vi "Realsense Cam Stream Restart.vi"(8 "error in (no error)":errorcluster, 10 "Stream Config":T1={"Stream Type"=enum."Color", "Resolution"=27} {"Resolution" items=["424 x 240 @6fps", "424 x 240 @15fps", "424 x 240 @30fps", "424 x 240 @60fps", "424 x 240 @90fps", "480 x 270 @6fps", "480 x 270 @15fps", "480 x 270 @30fps", "480 x 270 @60fps", "480 x 270 @90fps", "640 x 360 @6fps", "640 x 360 @15fps", "640 x 360 @30fps", "640 x 360 @60fps", "640 x 360 @90fps", "640 x 480 @6fps", "640 x 480 @15fps", "640 x 480 @30fps", "640 x 480 @60fps", "640 x 480 @90fps", "848 x 100 @100fps", "848 x 480 @6fps", "848 x 480 @15fps", "848 x 480 @30fps", "848 x 480 @60fps", "848 x 480 @90fps", "1280 x 720 @6fps", "1280 x 720 @15fps", "1280 x 720 @30fps", "1280 x 800 @15fps", "1280 x 800 @30fps"]}, 11 "Realsense Cam in":refnum<class "Realsense Cam.lvclass">) -> (0 "error out":errorcluster, 3 "Realsense Cam out":refnum<class "Realsense Cam.lvclass">)   [LabVIEW 2018, in "Realsense Cam.lvclass"]
uses:
  Realsense Cam.lvclass
  Private/Stream Config STYP.ctl
  Private/Stream Types Enum STYP.ctl
  Realsense Cam.lvclass/Realsense Cam.ctl
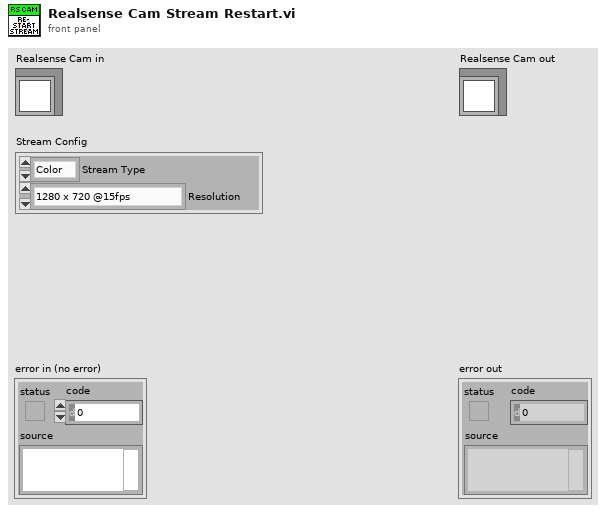
[diagram p1: front panel]
types:
  T1 = typedef "Realsense Cam.lvclass/Stream Config STYP.ctl" = cluster{"Stream Type":T2, "Resolution":u16}
  T2 = typedef "Realsense Cam.lvclass/Stream Types Enum STYP.ctl" = enum16{"Depth", "Left IR", "Left IR Unrectified", "Right IR", "Right IR Unrectified", "Color", "RGB Ext."}
  T3 = cluster{"Depth?":bool, "Left IR?":bool, "Left IR Unrectified?":bool, "Right IR?":bool, "Right IR Unrectified?":bool, "Color?":bool, "RGB Ext.?":bool}
  T4 = typedef "Realsense Cam.lvclass/Activated Stream STYP.ctl" = cluster{"Stream Config":T1, "Profile Handle":u64, "Stream":T5}
  T5 = typedef "Realsense Cam.lvclass/Stream STYP.ctl" = cluster{"Strings":string[], "Intrinsics":cluster{"width":i32, "height":i32, "fps":i32, "Profile":u64, "ppx":sgl, "ppy":sgl, "fx":sgl, "fy":sgl, "model":u32}[], "Current Data":T6}
  T6 = typedef "Realsense Cam.lvclass/Stream Frame Data STYP.ctl" = cluster{"Depths":sgl[][], "Bytes":u8[], "16-Bit IR":u16[], "Height":i32, "Width":i32}
  T7 = cluster{"Status[0]":bool, "Status[1]":bool, "Status[2]":bool, "Status[3]":bool, "Status[4]":bool, "Status[5]":bool, "Status[6]":bool}
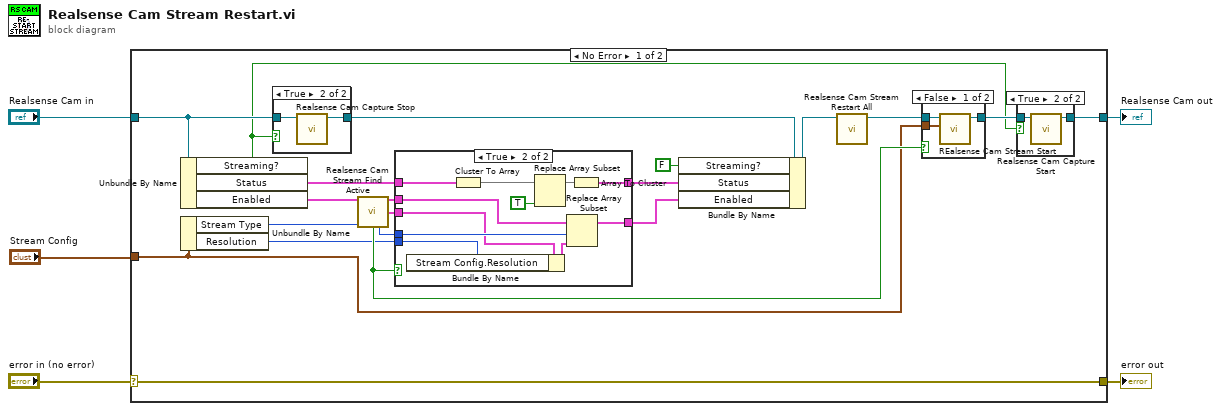
[diagram p0: block diagram]
diagram:
  n1 = case shown="No Error" "error in (no error)" {
    selector: "error in (no error)" -> [w24 w49]
    tunnel: [w24 w49] -> w4
    tunnel: [w7 w48] -> w2
    tunnel: "Realsense Cam in" -> [w19 w48]
    tunnel: "Stream Config" -> [w9 _]
    frame No Error {
      n2 = Unbundle By Name(w19) -> ("Streaming?"=w6:bool, "Status"=w23:T3, "Enabled"=w21:T4[])
      n3 = Unbundle By Name(w9) -> ("Stream Type"=w12:T2, "Resolution"=w11:u16)
      n4 = case shown="True" w6 {
        tunnel: w19 -> [w32 w34]
        tunnel: [w32 w33] -> w16
        frame False {
        }
        frame True {
          n5 = call-dynamic "Realsense Cam Capture Stop.vi"("Realsense Cam in"=w34) -> ("Realsense Cam out"=w33:refnum<class "Realsense Cam.lvclass">)  [unwired: 8 in, 2 out]
        }
      }
      n6 = call "Realsense Cam Stream Find Active.vi"("Streams"=w21, "Stream Types"=w12) -> ("Activated Stream"=w22:T4, "Found?"=w17:bool, "Index"=w20:i32)  [unwired: 11 in]
      n7 = case shown="True" w17 {
        tunnel: w23 -> [w36 w47]
        tunnel: w22 -> [_ w39]
        tunnel: w21 -> [w35 w43]
        tunnel: w20 -> [_ w42]
        tunnel: [w36 w41] -> w14
        tunnel: [w35 w40] -> w10
        tunnel: w11 -> [_ w37]
        frame False {
        }
        frame True {
          n8 = Bundle By Name(cluster=w39, "Stream Config.Resolution"=w37) -> (w38:T4)
          n9 = Cluster To Array(cluster=w47) -> (array=w46:bool[])
          n10 = Replace Array Subset(array=w46, new element=TRUE ("new element/subarray")) -> (w44:bool[])  [unwired: 1 in]
          n11 = Replace Array Subset(array=w43, new element=w38, index=w42) -> (w40:T4[])
          n12 = Array To Cluster(array=w44) -> (cluster=w41:T7)
        }
      }
      n13 = Bundle By Name(cluster=w16, "Streaming?"=FALSE ("Stream Data.Started?"), "Status"=w14, "Enabled"=w10) -> (w15:refnum<class "Realsense Cam.lvclass">)
      n14 = call-dynamic "Realsense Cam Stream Restart All.vi"("Realsense Cam in"=w15) -> ("Realsense Cam out"=w18:refnum<class "Realsense Cam.lvclass">)  [unwired: 9 in, 1 out]
      n15 = case shown="False" w17 {
        tunnel: [w30 w31] -> w8
        tunnel: w18 -> [w29 w31]
        tunnel: w9 -> [w28 _]
        frame False {
          n16 = call-dynamic "REalsense Cam Stream Start.vi"("Stream Config"=w28, "Realsense Cam in"=w29) -> ("Realsense Cam out"=w30:refnum<class "Realsense Cam.lvclass">)  [unwired: 8 in, 1 out]
        }
        frame True {
        }
      }
      n17 = case shown="True" w6 {
        tunnel: w8 -> [w25 w27]
        tunnel: [w25 w26] -> w7
        frame False {
        }
        frame True {
          n18 = call-dynamic "Realsense Cam Capture Start.vi"("Realsense Cam in"=w27) -> ("Realsense Cam out"=w26:refnum<class "Realsense Cam.lvclass">)  [unwired: 8 in, 2 out]
        }
      }
    }
    frame Error {
    }
  }
  "error out" <- w4
  "Realsense Cam out" <- w2
